vi "Configure Internal Trigger Rate [IT].vi"(8 "error in (no error)":errorcluster, 9 "trigger rate (0.0 trig/sec)":dbl[unit] format="%.3f", 11 "CS++Fgen in":refnum<class "CS++Fgen.lvclass">) -> (0 "error out":errorcluster, 3 "CS++Fgen out":refnum<class "CS++Fgen.lvclass">)   [LabVIEW 2013, in "CS++Fgen.lvlib" / "CS++Fgen.lvclass"]
doc: "This VI configures the rate at which the function generator's internal trigger source generates trigger signals.\n\nNotes:\n\n(1) This VI is part of the IviFgenInternalTrigger [IT] extension group."
uses:
  CS++Fgen.lvclass
  Core/Classes/CS++ProcessVariables/ProcessVariable/PV.lvclass
  Core/Classes/CS++ProcessVariables/ProcessVariable/PV.lvclass/PV.ctl
  CS++Fgen.lvclass/CS++Fgen.ctl
  Core/Classes/CS++ProcessVariables/PVConnection/PVConnection.lvclass
  Core/Classes/CS++ProcessVariables/ProcessVariable/Write Data.vi
  Core/Classes/CS++ProcessVariables/ProcessVariable/Write Timestamp.vi
  Core/Classes/CS++ProcessVariables/ProcessVariable/Write Quality.vi
  Core/Classes/CS++ProcessVariables/ProcessVariable/Write status.vi
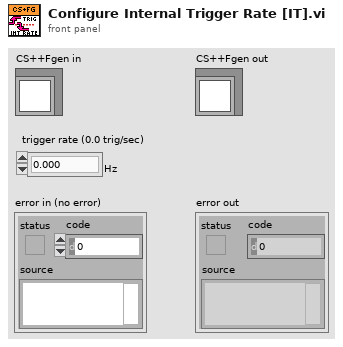
[diagram p1: front panel]
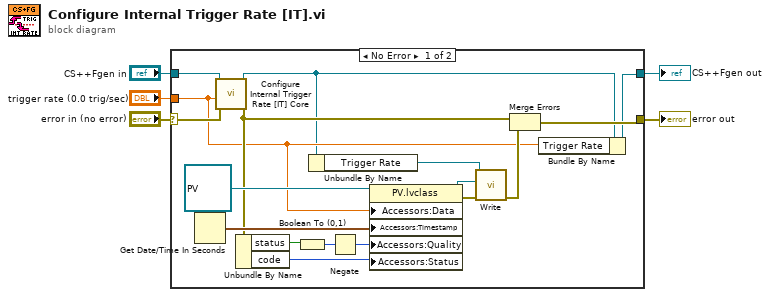
[diagram p0: block diagram]
diagram:
  n1 = case shown="No Error" "error in (no error)" {
    selector: "error in (no error)" -> [w21 w24]
    tunnel: [w9 w24] -> w4
    tunnel: [w7 w23] -> w2
    tunnel: "CS++Fgen in" -> [w22 w23]
    tunnel: "trigger rate (0.0 trig/sec)" -> [w10 _]
    frame No Error {
      n2 = Get Date/Time In Seconds() -> (seconds since 1Jan1904=w20:timestamp)
      n3 = call-dynamic "Configure Internal Trigger Rate [IT] Core.vi"("error in (no error)"=w21, "trigger rate (0.0 trig/sec)"=w10, "CS++Fgen in"=w22) -> ("error out"=w11:errorcluster, "CS++Fgen out"=w8:refnum<class "CS++Fgen.lvclass">)  [unwired: 7 in]
      n4 = Unbundle By Name(w11) -> ("status"=w15:bool, "code"=w13:i32)
      n5 = Boolean To (0,1)(Boolean=w15) -> (0, 1=w14:i16)
      n6 = Unbundle By Name(w8) -> ("Trigger Rate"=w6:refnum<class "PVConnection.lvclass">)
      n7 = Negate(x=w14) -> (-x=w12:i16)
      n8 = property class="PV.lvclass"(reference=refnum<class "PV.lvclass"> refnum ("PV"), "Accessors:Data"=w10, "Accessors:Timestamp"=w20, "Accessors:Quality"=w12, "Accessors:Status"=w13) -> (reference out=w17:refnum<class "PV.lvclass">, error out=w18:errorcluster)  [unwired: 1 in]
      n9 = call-dynamic "Write.vi"("error in (no error)"=w18, "PV"=w17, "PVConnection in"=w6) -> ("error out"=w16:errorcluster)  [unwired: 7 in, 1 out]
      n10 = Merge Errors(w11, w16) -> (w9:errorcluster)
      n11 = Bundle By Name(cluster=w8, "Trigger Rate"=w10) -> (w7:refnum<class "CS++Fgen.lvclass">)
    }
    frame Error {
    }
  }
  "error out" <- w4
  "CS++Fgen out" <- w2
